vi "RT_Fourierseries.vi"() -> ()   [LabVIEW 2018]
panel:
  out "no. cycles":dbl
  in  "phase":dbl
  out "x,i":dbl[](array[numeric])=[5.5, 4.058601056159812, 0.9216218905270259, -1.3271440933602046, -0.8354860874339969, 1.9916385766070146, 4.825650181703828, 5.3322965367607935, 3.09427505830386, -0.0450532277586948, -1.4999600494850531, -0.072101889033922, 3.0624565424930745, 5.321915695033998, 4.845257262233128, 2.0250840792971476, -0.8157497695851905, -1.3373729076113228, 0.8898529739235752, 4.031458713112125, 5.4998401988522385, 4.085555418172324, 0.9534892791645411, -1.31661146114058, -0.8549634830363781, 1.9581938374397765, 4.805785077093263, 5.3423730900240125, 3.125993650451633, -0.0178178225674559, -1.4996404508376084, -0.09896133644620253, 3.030541008525172, 5.311231512769584, 4.864604528261745, 2.058527291436042, -0.7957563317106686, -1.3472969698503645, 0.8581854303309544, 4.004130867530732, 5.499360810001185, 4.112319337813647, 0.9854522298673911, -1.3057759727391347, -0.8741801778151137, 1.9247529157998269, 4.785663762382315, 5.352144434683785, 3.1576094225549762, 0.009601839540371637, -1.4990012827268502, -0.12562911732667503, 2.9985313707652828, 5.300244965593036, 4.883690213095237, 2.091965159158726, -0.7755075995100604, -1.3569153738621518, 0.8266221514690681, 3.976620014856264, 5.498561877222205, 4.138890371138071, 1.0175078239405875, -1.2946386175978768, -0.8931344169988118, 1.8913188653429627, 4.765288074947627, 5.361609678470338, 3.1891194876215403, 0.03720325473992836, -1.4980426035183774, -0.1521027965084727, 2.966430552171596, 5.288957056740248, 4.90251257392539, 2.125394629088274, -0.7550054219951385, -1.3662272413426924, 0.795166019536846, 3.948928667240618, 5.497443473469799, 4.165266091813233, 1.0496531342294175, -1.2832004127237315, -0.9118244697822577, 1.8578947390975602, 4.744659875393928, 5.370767957065493, 3.220520968311609, 0.06498390260960862, -1.496764500753927, -0.1783799565491755, 2.9342414840285698, 5.277368816965979, 4.9210698919894105, 2.158812648614642, -0.7342516713211058, -1.3752317219793513, 0.7638199069491849, 3.92105935331754]
  out "Time period":dbl=0.6666666666666666
  in  "frequency":dbl=1.5
  out "delt,i":dbl[](array[numeric])=[0.0, 0.1, 0.2, 0.30000000000000004, 0.4, 0.5, 0.6000000000000001, 0.7000000000000001, 0.8, 0.9, 1.0, 1.1, 1.2000000000000002, 1.3, 1.4000000000000001, 1.5, 1.6, 1.7000000000000002, 1.8, 1.9000000000000001, 2.0, 2.1, 2.2, 2.3000000000000003, 2.4000000000000004, 2.5, 2.6, 2.7, 2.8000000000000003, 2.9000000000000004, 3.0, 3.1, 3.2, 3.3000000000000003, 3.4000000000000004, 3.5, 3.6, 3.7, 3.8000000000000003, 3.9000000000000004, 4.0, 4.1000000000000005, 4.2, 4.3, 4.4, 4.5, 4.6000000000000005, 4.7, 4.800000000000001, 4.9, 5.0, 5.1000000000000005, 5.2, 5.300000000000001, 5.4, 5.5, 5.6000000000000005, 5.7, 5.800000000000001, 5.9, 6.0, 6.1000000000000005, 6.2, 6.300000000000001, 6.4, 6.5, 6.6000000000000005, 6.7, 6.800000000000001, 6.9, 7.0, 7.1000000000000005, 7.2, 7.300000000000001, 7.4, 7.5, 7.6000000000000005, 7.7, 7.800000000000001, 7.9, 8.0, 8.1, 8.200000000000001, 8.3, 8.4, 8.5, 8.6, 8.700000000000001, 8.8, 8.9, 9.0, 9.1, 9.200000000000001, 9.3, 9.4, 9.5, 9.600000000000001, 9.700000000000001, 9.8, 9.9]
  out "N":i32=100
  in  "amplitude":dbl=3.5 format="%#_13g"
  in  "offset":dbl=2.0
  out "computed amplitude":dbl=3.499099905625707
  out "b":dbl=0.08361292365301659
  in  "del t":dbl=0.1
  out "a":dbl=3.498100774498646
  out "simulated sine":cluster{dbl[], "delt,i":dbl[]}(graph)={[0.0, 0.1, 0.2, 0.30000000000000004, 0.4, 0.5, 0.6000000000000001, 0.7000000000000001, 0.8, 0.9, 1.0, 1.1, 1.2000000000000002, 1.3, 1.4000000000000001, 1.5, 1.6, 1.7000000000000002, 1.8, 1.9000000000000001, 2.0, 2.1, 2.2, 2.3000000000000003, 2.4000000000000004, 2.5, 2.6, 2.7, 2.8000000000000003, 2.9000000000000004, 3.0, 3.1, 3.2, 3.3000000000000003, 3.4000000000000004, 3.5, 3.6, 3.7, 3.8000000000000003, 3.9000000000000004, 4.0, 4.1000000000000005, 4.2, 4.3, 4.4, 4.5, 4.6000000000000005, 4.7, 4.800000000000001, 4.9, 5.0, 5.1000000000000005, 5.2, 5.300000000000001, 5.4, 5.5, 5.6000000000000005, 5.7, 5.800000000000001, 5.9, 6.0, 6.1000000000000005, 6.2, 6.300000000000001, 6.4, 6.5, 6.6000000000000005, 6.7, 6.800000000000001, 6.9, 7.0, 7.1000000000000005, 7.2, 7.300000000000001, 7.4, 7.5, 7.6000000000000005, 7.7, 7.800000000000001, 7.9, 8.0, 8.1, 8.200000000000001, 8.3, 8.4, 8.5, 8.6, 8.700000000000001, 8.8, 8.9, 9.0, 9.1, 9.200000000000001, 9.3, 9.4, 9.5, 9.600000000000001, 9.700000000000001, 9.8, 9.9], "delt,i"=[5.5, 4.058601056159812, 0.9216218905270259, -1.3271440933602046, -0.8354860874339969, 1.9916385766070146, 4.825650181703828, 5.3322965367607935, 3.09427505830386, -0.0450532277586948, -1.4999600494850531, -0.072101889033922, 3.0624565424930745, 5.321915695033998, 4.845257262233128, 2.0250840792971476, -0.8157497695851905, -1.3373729076113228, 0.8898529739235752, 4.031458713112125, 5.4998401988522385, 4.085555418172324, 0.9534892791645411, -1.31661146114058, -0.8549634830363781, 1.9581938374397765, 4.805785077093263, 5.3423730900240125, 3.125993650451633, -0.0178178225674559, -1.4996404508376084, -0.09896133644620253, 3.030541008525172, 5.311231512769584, 4.864604528261745, 2.058527291436042, -0.7957563317106686, -1.3472969698503645, 0.8581854303309544, 4.004130867530732, 5.499360810001185, 4.112319337813647, 0.9854522298673911, -1.3057759727391347, -0.8741801778151137, 1.9247529157998269, 4.785663762382315, 5.352144434683785, 3.1576094225549762, 0.009601839540371637, -1.4990012827268502, -0.12562911732667503, 2.9985313707652828, 5.300244965593036, 4.883690213095237, 2.091965159158726, -0.7755075995100604, -1.3569153738621518, 0.8266221514690681, 3.976620014856264, 5.498561877222205, 4.138890371138071, 1.0175078239405875, -1.2946386175978768, -0.8931344169988118, 1.8913188653429627, 4.765288074947627, 5.361609678470338, 3.1891194876215403, 0.03720325473992836, -1.4980426035183774, -0.1521027965084727, 2.966430552171596, 5.288957056740248, 4.90251257392539, 2.125394629088274, -0.7550054219951385, -1.3662272413426924, 0.795166019536846, 3.948928667240618, 5.497443473469799, 4.165266091813233, 1.0496531342294175, -1.2832004127237315, -0.9118244697822577, 1.8578947390975602, 4.744659875393928, 5.370767957065493, 3.220520968311609, 0.06498390260960862, -1.496764500753927, -0.1783799565491755, 2.9342414840285698, 5.277368816965979, 4.9210698919894105, 2.158812648614642, -0.7342516713211058, -1.3752317219793513, 0.7638199069491849, 3.92105935331754]}
  # "datapoints"
  # "sampling interval (s)"
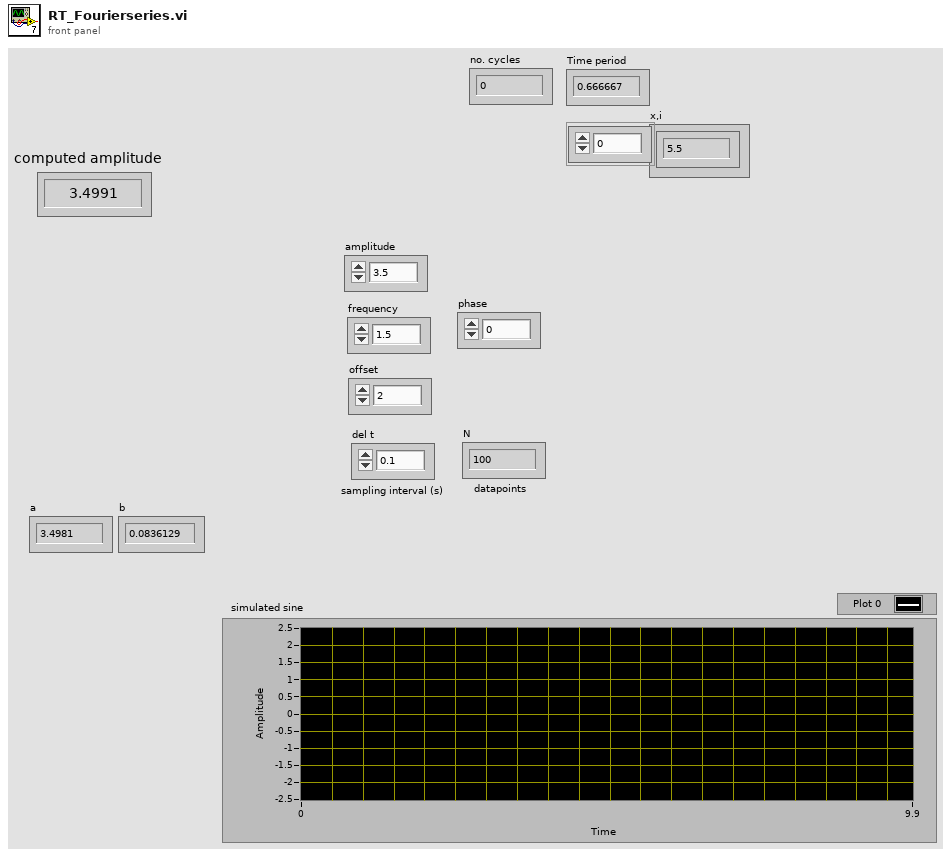
[diagram p1: front panel]
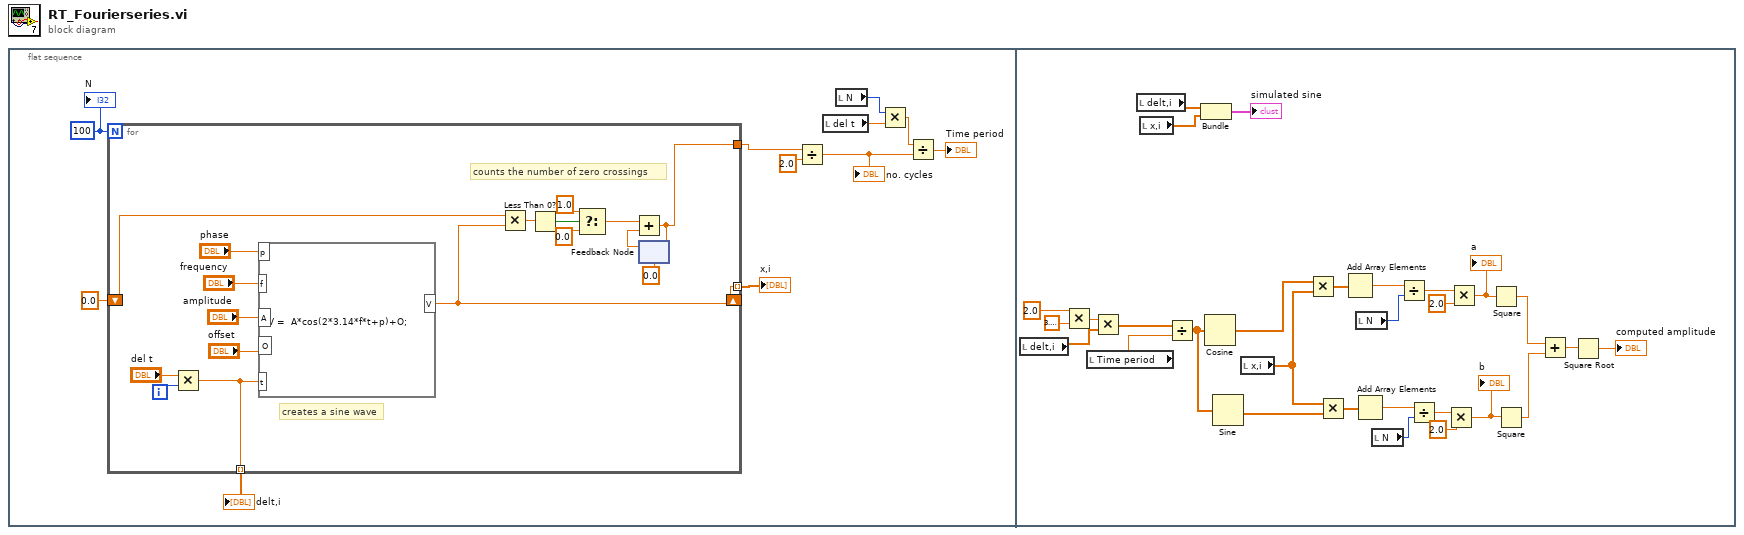
[diagram p0: block diagram]
diagram:
  n1 = flat-sequence {
    frame #0 {
      w10 = 100
      n2 = for {
        N: w10 -> [_]
        tunnel: [w16] -> w3 mode=indexing
        tunnel: [w26] -> w11 mode=indexing
        shift-right: [w16] -> _
        shift-left: 0.0 ("V") -> [w15]
        tunnel: [w17] -> w1
        i -> [w27]
        # "counts the number of zero crossings"
        # "creates a sine wave"
        n3 = Multiply(x="del t", y=w27) -> (x*y=w26:dbl)
        n4 = formula code="V =  A*cos(2*3.14*f*t+p)+O;"("A"="amplitude", "t"=w26, "O"="offset", "f"="frequency", "p"="phase") -> ("V"=w16:dbl)
        n5 = Multiply(x=w15, y=w16) -> (x*y=w25:dbl)
        n6 = Less Than 0?(x=w25) -> (x < 0?=w24:bool)
        n7 = Select(t=1.0, s=w24, f=0.0) -> (s? t:f=w21:dbl)
        n8 = feedback #1(0.0) -> (w20:dbl)
        n9 = Add(x=w21, y=w20) -> (x+y=w17:dbl)
        n10 = feedback-in #1(w17) -> ()
      }
      "delt,i" <- w11
      "x,i" <- w3
      n11 = Divide(x=w1, y=2.0) -> (x/y=w4:dbl)
      "no. cycles" <- w4
      n12 = local read "del t"() -> (w6:dbl)
      n13 = local read "N"() -> (w7:i32)
      n14 = Multiply(x=w7, y=w6) -> (x*y=w5:dbl)
      n15 = Divide(x=w5, y=w4) -> (x/y=→"Time period":dbl)
      "N" <- w10
    }
    frame #1 {
      n16 = local read "delt,i"() -> (w48:dbl[])
      n17 = Multiply(x=2.0, y=3.141592653589793) -> (x*y=w33:dbl)
      n18 = local read "Time period"() -> (w51:dbl)
      n19 = Multiply(x=w33, y=w48) -> (x*y=w34:dbl[])
      n20 = local read "delt,i"() -> (w50:dbl[])
      n21 = local read "x,i"() -> (w55:dbl[])
      n22 = Divide(x=w34, y=w51) -> (x/y=w38:dbl[])
      n23 = Bundle("delt,i"=w50, "x,i"=w55) -> (→"simulated sine":cluster{"delt,i":dbl[], "x,i":dbl[]})  [unwired: 1 in]
      n24 = Cosine(x=w38) -> (cos(x)=w57:dbl[])
      n25 = Sine(x=w38) -> (sin(x)=w54:dbl[])
      n26 = local read "x,i"() -> (w56:dbl[])
      n27 = Multiply(x=w57, y=w56) -> (x*y=w35:dbl[])
      n28 = Multiply(x=w56, y=w54) -> (x*y=w39:dbl[])
      n29 = Add Array Elements(numeric array=w35) -> (sum=w36:dbl)
      n30 = Add Array Elements(numeric array=w39) -> (sum=w40:dbl)
      n31 = local read "N"() -> (w52:i32)
      n32 = local read "N"() -> (w53:i32)
      n33 = Divide(x=w36, y=w52) -> (x/y=w37:dbl)
      n34 = Divide(x=w40, y=w53) -> (x/y=w41:dbl)
      n35 = Multiply(x=w41, y=2.0) -> (x*y=w43:dbl)
      "b" <- w43
      n36 = Multiply(x=w37, y=2.0) -> (x*y=w42:dbl)
      "a" <- w42
      n37 = Square(x=w42) -> (x^2=w44:dbl)
      n38 = Square(x=w43) -> (x^2=w45:dbl)
      n39 = Add(x=w44, y=w45) -> (x+y=w46:dbl)
      n40 = Square Root(x=w46) -> (sqrt(x)=→"computed amplitude":dbl)
    }
  }
